vi "Construct Mock Notification Msg.vi"(8 "error in (no error)":errorcluster) -> (0 "error out":errorcluster, 2 "Data leak test queue":refnum<queue>, 3 "MockNotificationMsg out":refnum<class "MockNotificationMsg.lvclass">)   [LabVIEW 2017, in "MockNotificationMsg.lvclass"]
uses:
  MockNotificationMsg.lvclass
  MockNotificationMsg.lvclass/MockNotificationMsg.ctl
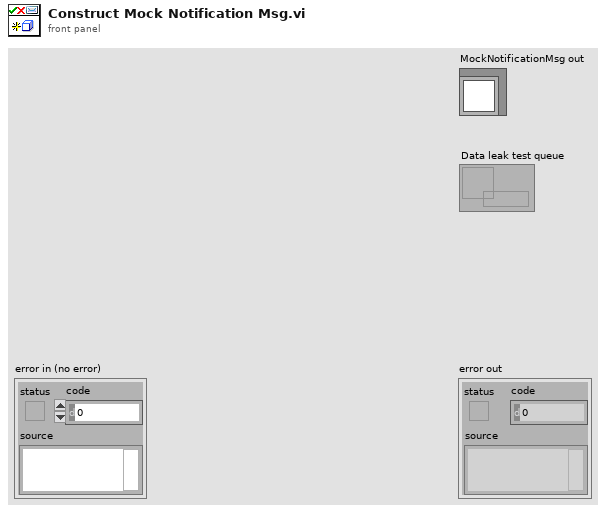
[diagram p1: front panel]
types:
  T1 = cluster{"Datum Name":string, "Value":variant, "Publication Time":timestamp}
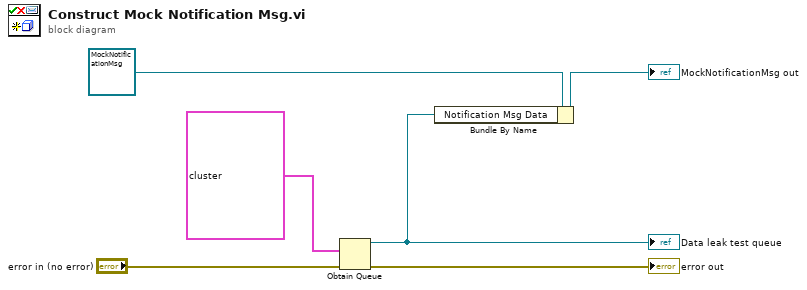
[diagram p0: block diagram]
diagram:
  n1 = Obtain Queue(element data type=T1 {"Datum Name"="", "Value"=variant, "Publication Time"=timestamp(0 s since 1904-01-01)}, error in (no error)="error in (no error)") -> (queue out=w1:refnum<queue>, error out=→"error out":errorcluster)  [unwired: 3 in, 1 out]
  "Data leak test queue" <- w1
  n2 = Bundle By Name(cluster=refnum<class "MockNotificationMsg.lvclass"> refnum ("MockNotificationMsg in"), "Notification Msg Data"=w1) -> (→"MockNotificationMsg out":refnum<class "MockNotificationMsg.lvclass">)
